vi "EnviraCom Communication Main.vi"() -> ()   [LabVIEW 2023]
panel:
  in  "ON (True), OFF (False)":bool
  in  "Boolean":bool
  out "Read Data":string
  in  "stop":bool
  in  "error in (no error)":errorcluster
  out "error out":errorcluster
  in  "VISA resource name":refnum<visa-resource-name>
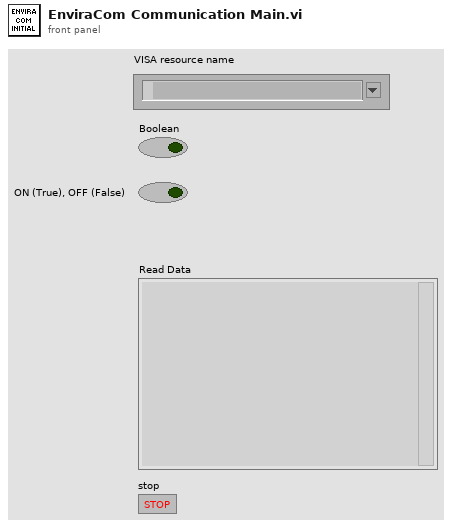
[diagram p1: front panel]
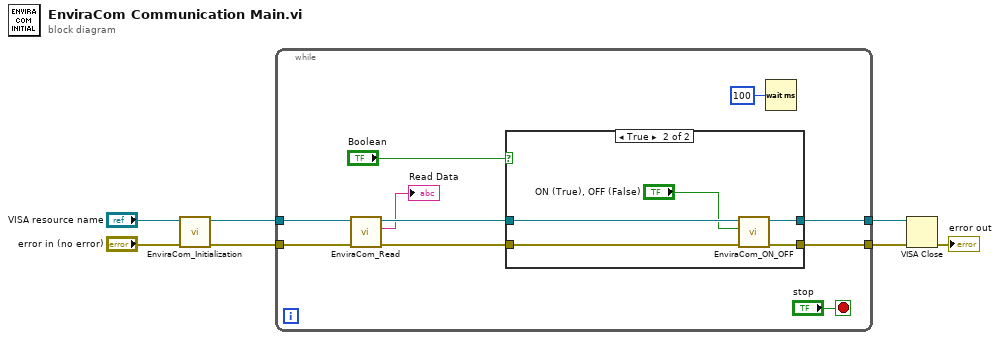
[diagram p0: block diagram]
diagram:
  n1 = call "EnviraCom_Initialization.vi"("error in (no error)"="error in (no error)", "VISA Refnum in"="VISA resource name") -> ("error out"=w4:errorcluster, "VISA Refnum out"=w5:refnum<visa-resource-name>)  [unwired: 8 in]
  n2 = while {
    tunnel: w5 -> [w17]
    tunnel: w4 -> [w16]
    tunnel: [w12] -> w3
    tunnel: [w10] -> w2
    stop <- "stop" stop-if-true
    n3 = call "EnviraCom_Read.vi"("error in (no error)"=w16, "VISA Refnum in"=w17) -> ("error out"=w13:errorcluster, "Read Data"=→"Read Data":string, "VISA Refnum out"=w11:refnum<visa-resource-name>)  [unwired: 7 in]
    n4 = case shown="True" "Boolean" {
      tunnel: w13 -> [w19 w24]
      tunnel: [w19 w23] -> w12
      tunnel: w11 -> [w18 w22]
      tunnel: [w18 w21] -> w10
      frame False {
      }
      frame True {
        n5 = call "EnviraCom_ON_OFF.vi"("error in (no error)"=w24, "ON (True), OFF (False)"="ON (True), OFF (False)", "VISA Refnum in"=w22) -> ("error out"=w23:errorcluster, "VISA Refnum out"=w21:refnum<visa-resource-name>)  [unwired: 7 in]
      }
    }
    n6 = Wait (ms)(milliseconds to wait=u32 100) -> ()  [unwired: 1 out]
  }
  n7 = VISA Close(VISA resource name=w2, error in (no error)=w3) -> (error out=→"error out":errorcluster)
